vi "Apply Transparency.vi"(9 "rect":T1, 11 "in":picture) -> (3 "out":picture)   [LabVIEW 2017, in "lv_icon.lvlib"]
doc: "Apply the magic transparent color to the glyph."
uses:
  <vilib>/LabVIEW Icon API/lv_icon/lv_icon.lvlib
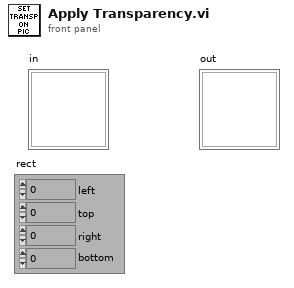
[diagram p1: front panel]
types:
  T1 = cluster{"left":i16, "top":i16, "right":i16, "bottom":i16}
  T2 = typedef "imagedata.ctl" = cluster{"image type":i32, "image depth":i32, "image":u8[], "mask":u8[], "colors":u32[], "Rectangle":cluster{"left":i16, "top":i16, "right":i16, "bottom":i16}}
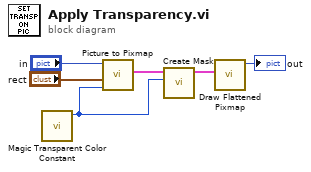
[diagram p0: block diagram]
diagram:
  n1 = call <vilib>:"Magic Transparent Color Constant.vi"() -> ("Magic transparent color constant"=w1:u32)  [unwired: 11 out]
  n2 = call <vilib>:"Picture to Pixmap.vi"("Background Color"=w1, "rect"="rect", "picture"="in") -> ("image data"=w6:T2)  [unwired: 1 in, 7 out]
  n3 = call <vilib>:"Create Mask.vi"("Mask Color (Black)"=w1, "image data"=w6) -> ("image data"=w5:T2)  [unwired: 2 in, 7 out]
  n4 = call <vilib>:"Draw Flattened Pixmap.vi"("image data"=w5) -> ("new picture"=→"out":picture)  [unwired: 1 in, 7 out]
